vi "Device Sorter.vi"(0 "Mercury Ref":T3, 5 "Devices":string[](array[string]), 11 "error in":errorcluster, 12 "ISOBUS address":T2=-1) -> (1 "Temp Dev Settings Array":T6[](array[typedef]), 2 "Heater Device Settings Array":T15[](array[typedef]), 3 "Aux Device Settings Array":T17[](array[typedef]) {"Signals"."% Open" min=0.0 max=100.0 step=0.1 format="%.4f"; "Signals"."Position" max=20.0 step=1.0 format="%.4f"; "Speed" max=7 step=1; "Gear" max=7 step=1; "Temp V Err" min=0.0 max=20.0 step=0.1; "Temp Err" min=0.0 max=20.0 step=0.1; "Scaling Factor" min=0.0 max=99.0 step=0.1; "Min Flow" min=0.0 max=20.0 step=0.1}, 4 "Mercury Ref Out":T3, 6 "Device_ref_Array":T3[](array[typedef]), 8 "Ch_type_index":i32[](array[numeric]), 10 "Device_Present?":bool[](array[boolean]), 13 "Level Device Settings Array":T19[](array[typedef]), 14 "Pressure Device Settings Array":T27[](array[typedef]), 15 "error out":errorcluster)   [LabVIEW 2013]
uses:
  <instrlib>/Mercury iXX/Public/Controls/Mercury Reference.ctl
  <instrlib>/Mercury iXX/Public/Controls/Comms Transport Layer.ctl
  <instrlib>/Mercury iXX/Private/Controls/Query Dynamic Reference.ctl
  <instrlib>/Mercury iXX/Public/Libraries/Temperature/Controls/Temperature Device (Read).ctl
  <instrlib>/Mercury iXX/Public/Controls/Manufacturing Data.ctl
  <instrlib>/Mercury iXX/Public/Libraries/Temperature/Controls/Temperature Sensor Type.ctl
  <instrlib>/Mercury iXX/Public/Libraries/Temperature/Controls/Excitation Cluster.ctl
  <instrlib>/Mercury iXX/Public/Libraries/Temperature/Controls/Excitation Type.ctl
  <instrlib>/Mercury iXX/Public/Libraries/Temperature/Controls/Calibration Cluster.ctl
  <instrlib>/Mercury iXX/Public/Libraries/Temperature/Controls/Calibration Interpolation.ctl
  <instrlib>/Mercury iXX/Public/Libraries/Temperature/Controls/Loop Cluster.ctl
  <instrlib>/Mercury iXX/Public/Libraries/Temperature/Controls/Temperature Signals Cluster.ctl
  <instrlib>/Mercury iXX/Public/Libraries/Heater/Controls/Heater Device (Read).ctl
  <instrlib>/Mercury iXX/Public/Libraries/Heater/Controls/Heater Signals Cluster.ctl
  <instrlib>/Mercury iXX/Public/Libraries/Auxiliary/Controls/AUX Device (Read).ctl
  <instrlib>/Mercury iXX/Public/Libraries/Auxiliary/Controls/AUX Signals (Read).ctl
  <instrlib>/Mercury iXX/Public/Libraries/Level Meter/Controls/Level Meter (Read).ctl
  <instrlib>/Mercury iXX/Public/Libraries/Level Meter/Controls/Nitrogen Configuration.ctl
  <instrlib>/Mercury iXX/Public/Libraries/Level Meter/Controls/Frequency Configuration.ctl
  <instrlib>/Mercury iXX/Public/Libraries/Level Meter/Controls/Signals.ctl
  <instrlib>/Mercury iXX/Public/Libraries/Level Meter/Controls/Helium Configuration.ctl
  <instrlib>/Mercury iXX/Public/Libraries/Level Meter/Controls/Resistance Configuration.ctl
  <instrlib>/Mercury iXX/Public/Libraries/Level Meter/Controls/Pre-Pulse.ctl
  <instrlib>/Mercury iXX/Public/Libraries/Level Meter/Controls/Pulse.ctl
  <instrlib>/Mercury iXX/Public/Libraries/Pressure/Controls/Pressure Device (Read).ctl
  <instrlib>/Mercury iXX/Public/Libraries/Pressure/Controls/Pressure Sensor Type.ctl
  <instrlib>/Mercury iXX/Public/Libraries/Pressure/Controls/Calibration Cluster.ctl
  <instrlib>/Mercury iXX/Public/Libraries/Pressure/Controls/Calibration Interpolation.ctl
  <instrlib>/Mercury iXX/Public/Libraries/Pressure/Controls/Loop Cluster.ctl
  <instrlib>/Mercury iXX/Public/Libraries/Pressure/Controls/Pressure Signals Cluster.ctl
  <instrlib>/Mercury iXX/Public/Controls/ISOBus Address.ctl
  <instrlib>/Mercury iXX/Public/Libraries/Temperature/Open/Open Temperature Device.vi
  <instrlib>/Mercury iXX/Public/Libraries/Temperature/Configuration/Read/Temperature Device (Read).vi
  <instrlib>/Mercury iXX/Public/Libraries/Heater/Open/Open Heater Device.vi
  <instrlib>/Mercury iXX/Public/Libraries/Heater/Configuration/Read/Heater Device (Read).vi
  <instrlib>/Mercury iXX/Public/Libraries/Auxiliary/Open/Open Auxiliary Device.vi
  <instrlib>/Mercury iXX/Public/Libraries/Auxiliary/Configuration/Read/Aux Device (Read).vi
  <instrlib>/Mercury iXX/Public/Libraries/Level Meter/Open/Open Level Meter Device.vi
  <instrlib>/Mercury iXX/Public/Libraries/Level Meter/Configuration/Read/Level Meter Device (Read).vi
  <instrlib>/Mercury iXX/Public/Libraries/Pressure/Open/Open Pressure Device.vi
  <instrlib>/Mercury iXX/Public/Libraries/Pressure/Configuration/Read/Pressure Device (Read).vi
  <instrlib>/Mercury iXX/Mercury iXX.lvlib
  <instrlib>/Mercury iXX/Public/Libraries/Temperature.lvlib
  <instrlib>/Mercury iXX/Public/Libraries/Heater.lvlib
  <instrlib>/Mercury iXX/Public/Libraries/Auxiliary.lvlib
  <instrlib>/Mercury iXX/Public/Libraries/Level Meter.lvlib
  <instrlib>/Mercury iXX/Public/Libraries/Pressure.lvlib
panel:
  in  "Tab Control":T1(tab)
  in  "Pres Dev":T27
  in  "LVL Dev":T19
  in  "Aux Dev":T17 {"Signals"."% Open" min=0.0 max=100.0 step=0.1 format="%.4f"; "Signals"."Position" max=20.0 step=1.0 format="%.4f"; "Speed" max=7 step=1; "Gear" max=7 step=1; "Temp V Err" min=0.0 max=20.0 step=0.1; "Temp Err" min=0.0 max=20.0 step=0.1; "Scaling Factor" min=0.0 max=99.0 step=0.1; "Min Flow" min=0.0 max=20.0 step=0.1}
  in  "Htr Dev Det":T15
  in  "Device Det":T6
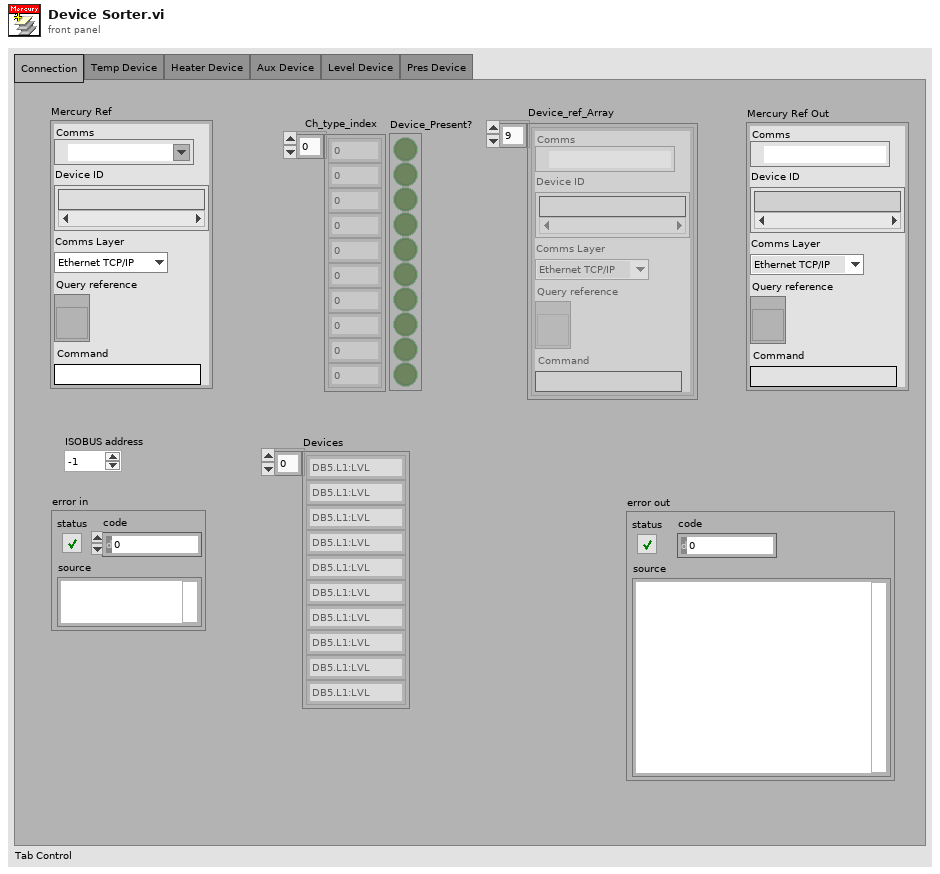
[diagram p1: front panel]
types:
  T1 = enum32{"Connection", "Temp Device", "Heater Device", "Aux Device", "Level Device", "Pres Device"}
  T2 = typedef "Mercury iXX.lvlib/ISOBus Address.ctl" = i32
  T3 = typedef "Mercury iXX.lvlib/Mercury Reference.ctl" = cluster{"Comms":refnum<visa-resource-name>, "Device ID":string[], "Comms Layer":T4, "Command":string, "Query reference":T5}
  T4 = typedef "Mercury iXX.lvlib/Comms Transport Layer.ctl" = enum16{"Ethernet TCP/IP", "USB", "ISOBus - RS-232", "GPIB"}
  T5 = typedef "Mercury iXX.lvlib/Query Dynamic Reference.ctl" = refnum<vi>
  T6 = typedef "Mercury iXX.lvlib/Temperature.lvlib/Temperature Device (Read).ctl" = cluster{"Manufacturing":T7, "Temperature Sensor Type":T8, "Excitation":T9, "Calibration":T11, "Control Loop":T13, "Temperature Signals":T14, "Nickname":string, "Status":string}
  T7 = typedef "Mercury iXX.lvlib/Manufacturing Data.ctl" = cluster{"Hardware Version":string, "Firmware Version":string, "Serial Number":string}
  T8 = typedef "Mercury iXX.lvlib/Temperature.lvlib/Temperature Sensor Type.ctl" = string
  T9 = typedef "Mercury iXX.lvlib/Temperature.lvlib/Excitation Cluster.ctl" = cluster{"Excitation Type":T10, "Magnitude":string}
  T10 = typedef "Mercury iXX.lvlib/Temperature.lvlib/Excitation Type.ctl" = string
  T11 = typedef "Mercury iXX.lvlib/Temperature.lvlib/Calibration Cluster.ctl" = cluster{"Filename":string, "Interpolation":T12, "Scaling Factor":string, "Offset Factor":string, "Hot Limit":string, "Cold Limit":string, "Last Calibration":string, "Reference":string}
  T12 = typedef "Mercury iXX.lvlib/Temperature.lvlib/Calibration Interpolation.ctl" = string
  T13 = typedef "Mercury iXX.lvlib/Temperature.lvlib/Loop Cluster.ctl" = cluster{"Heater":string, "Auxiliary":string, "Heater Auto":string, "Percentage Heat":string, "Temperature Set Point":string, "PID Auto (from file)":string, "P Value":string, "I Value":string, "D Value":string, "Auto PID Table Filename":string, "Flow Auto":string, "Target Heater Table":string, "Sweep mode":string, "Sweep Table Filename":string, "Percentage Flow":string}
  T14 = typedef "Mercury iXX.lvlib/Temperature.lvlib/Temperature Signals Cluster.ctl" = cluster{"Voltage":string, "Current":string, "Power":string, "Resistance":string, "Temperature":string, "Sensitivity":string, "Reference":string}
  T15 = typedef "Mercury iXX.lvlib/Heater.lvlib/Heater Device (Read).ctl" = cluster{"Manufacturing":T7, "Nickname":string, "Voltage Limit":string, "Nominal Resistance":string, "Maximum Power":string, "Heater Signals":T16, "Status":string}
  T16 = typedef "Mercury iXX.lvlib/Heater.lvlib/Heater Signals Cluster.ctl" = cluster{"Voltage":string, "Current":string, "Power":string}
  T17 = typedef "Mercury iXX.lvlib/Auxiliary.lvlib/AUX Device (Read).ctl" = cluster{"Manufacturing":T7, "Min Flow":dbl, "Scaling Factor":dbl, "Temp Err":dbl, "Temp V Err":dbl, "Gear":u32, "Speed":u32, "Signals":T18, "Nickname":string, "Status":string}
  T18 = typedef "Mercury iXX.lvlib/Auxiliary.lvlib/AUX Signals (Read).ctl" = cluster{"Position":dbl, "% Open":dbl, "I0":string, "I1":string, "I2":string, "I3":string, "O0":string, "O1":string, "O2":string, "O3":string}
  T19 = typedef "Mercury iXX.lvlib/Level Meter.lvlib/Level Meter (Read).ctl" = cluster{"Manufacturing":T7, "Nitrogen Configuration":T20, "Signals":T22, "Nickname":string, "Status":string, "Helium Configuration":T23}
  T20 = typedef "Mercury iXX.lvlib/Level Meter.lvlib/Nitrogen Configuration.ctl" = cluster{"Frequency Configuration":T21, "Pulse Period":dbl}
  T21 = typedef "Mercury iXX.lvlib/Level Meter.lvlib/Frequency Configuration.ctl" = cluster{"Freq 0%":dbl, "Freq 100%":dbl}
  T22 = typedef "Mercury iXX.lvlib/Level Meter.lvlib/Signals.ctl" = cluster{"Helium Signals":cluster{"Resistance":dbl, "Level":dbl}, "Nitrogen Signals":cluster{"Count":dbl, "Freq":dbl, "Level":dbl}}
  T23 = typedef "Mercury iXX.lvlib/Level Meter.lvlib/Helium Configuration.ctl" = cluster{"Resistance Configuration":T24, "Pre-Pulse":T25, "Pulse":T26}
  T24 = typedef "Mercury iXX.lvlib/Level Meter.lvlib/Resistance Configuration.ctl" = cluster{"Res 0%":dbl, "Res 100%":dbl}
  T25 = typedef "Mercury iXX.lvlib/Level Meter.lvlib/Pre-Pulse.ctl" = cluster{"Magnitude":dbl, "Duration":dbl}
  T26 = typedef "Mercury iXX.lvlib/Level Meter.lvlib/Pulse.ctl" = cluster{"Magnitude":dbl, "Duration":dbl, "Delay":dbl}
  T27 = typedef "Mercury iXX.lvlib/Pressure.lvlib/Pressure Device (Read).ctl" = cluster{"Manufacturing":T7, "Temperature Sensor Type":T28, "Calibration":T29, "Control Loop":T31, "Pressure Signals":T32, "Nickname":string, "Status":string}
  T28 = typedef "Mercury iXX.lvlib/Pressure.lvlib/Pressure Sensor Type.ctl" = string
  T29 = typedef "Mercury iXX.lvlib/Pressure.lvlib/Calibration Cluster.ctl" = cluster{"Filename":string, "Interpolation":T30, "Scaling Factor":string, "Offset Factor":string, "High Limit":string, "Low Limit":string, "Last Calibration":string}
  T30 = typedef "Mercury iXX.lvlib/Pressure.lvlib/Calibration Interpolation.ctl" = string
  T31 = typedef "Mercury iXX.lvlib/Pressure.lvlib/Loop Cluster.ctl" = cluster{"Heater":string, "Auxiliary":string, "Heater Auto":string, "Percentage Heat":string, "Pressure Set Point":string, "PID Auto (from file)":string, "P Value":string, "I Value":string, "D Value":string, "Auto PID Table Filename":string, "Flow Auto":string, "Target Heater Table":string, "Sweep mode":string, "Sweep Table Filename":string, "Percentage Flow":string}
  T32 = typedef "Mercury iXX.lvlib/Pressure.lvlib/Pressure Signals Cluster.ctl" = cluster{"Voltage":string, "Current":string, "Power":string, "Pressure":string}
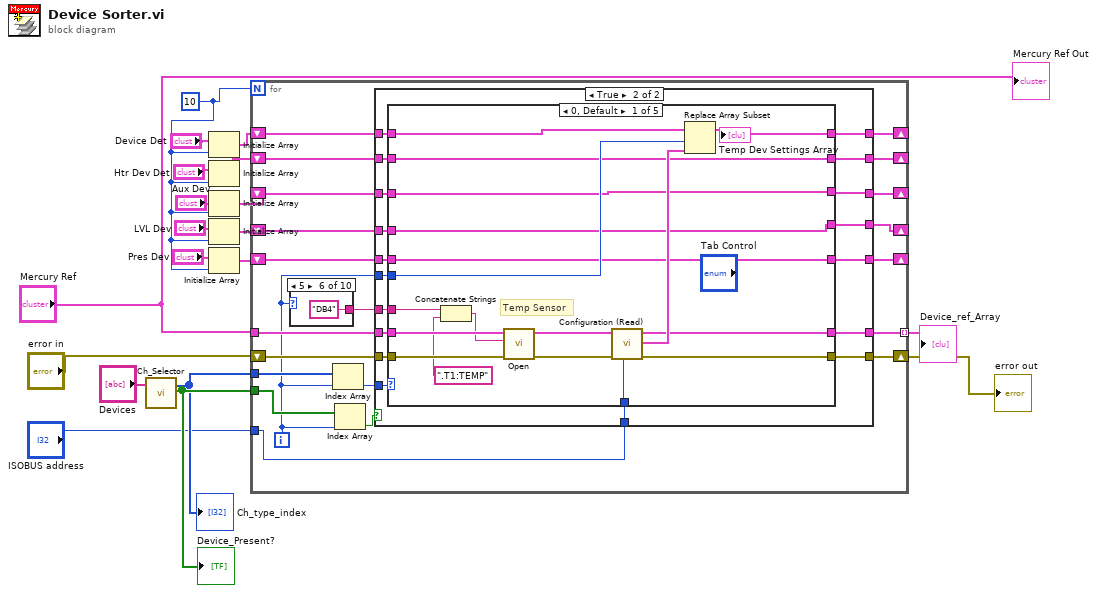
[diagram p0: block diagram]
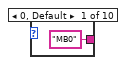
[diagram p2: hidden frame]
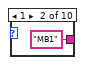
[diagram p3: hidden frame]
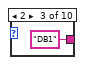
[diagram p4: hidden frame]
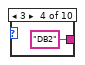
[diagram p5: hidden frame]
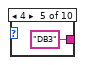
[diagram p6: hidden frame]
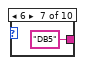
[diagram p7: hidden frame]
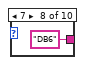
[diagram p8: hidden frame]
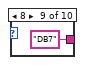
[diagram p9: hidden frame]
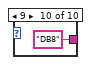
[diagram p10: hidden frame]
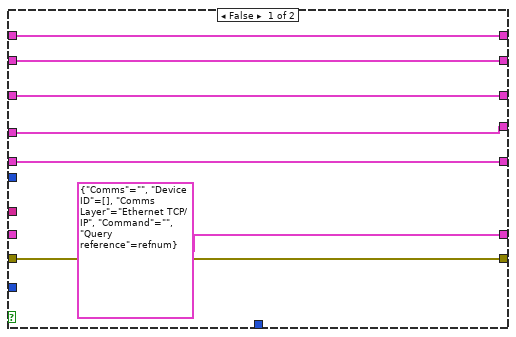
[diagram p11: hidden frame]
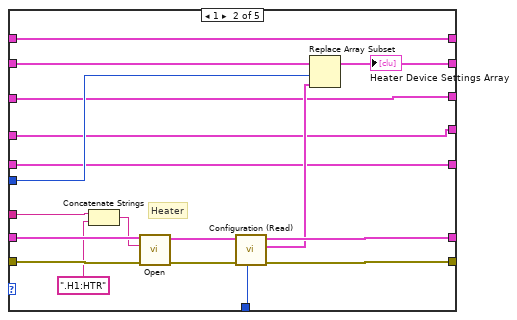
[diagram p12: hidden frame]
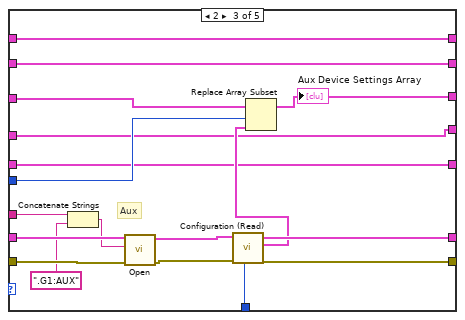
[diagram p13: hidden frame]
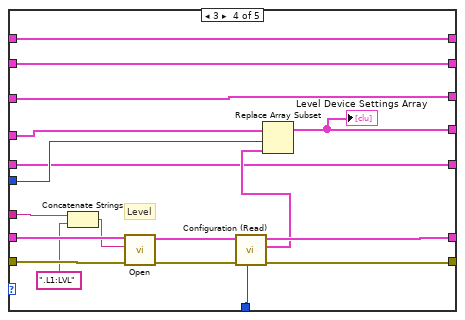
[diagram p14: hidden frame]
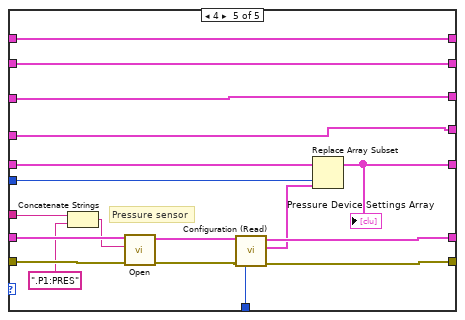
[diagram p15: hidden frame]
diagram:
  w9 = 10
  n1 = call <instrlib>:"Ch_Selector.vi"("Devices"="Devices") -> ("Ch_type_index"=w18:i32[], "Device_Present?"=w19:bool[])
  "Ch_type_index" <- w18
  "Device_Present?" <- w19
  n2 = Initialize Array("Device Det", w9) -> (w14:T6[])
  n3 = Initialize Array("Htr Dev Det", w9) -> (w12:T15[])
  n4 = Initialize Array("Aux Dev", w9) -> (w10:T17[])
  n5 = Initialize Array("LVL Dev", w9) -> (w7:T19[])
  n6 = Initialize Array("Pres Dev", w9) -> (w5:T27[])
  n7 = for {
    N: w9 -> [_]
    tunnel: "Mercury Ref" -> [w40]
    tunnel: [w39] -> w17 mode=indexing
    tunnel: w18 -> [w38]
    tunnel: w19 -> [w37]
    shift-right: [w32] -> w16
    shift-left: "error in" -> [w33]
    shift-right: [w30] -> _
    shift-left: w14 -> [w29]
    shift-right: [w28] -> _
    shift-left: w12 -> [w27]
    tunnel: "ISOBUS address" -> [w20]
    shift-right: [w26] -> _
    shift-left: w10 -> [w25]
    shift-right: [w23] -> _
    shift-left: w7 -> [w24]
    shift-right: [w22] -> _
    shift-left: w5 -> [w21]
    i -> [w31]
    n8 = case shown="5" w31 {
      tunnel: ["MB0" "MB1" "DB1" "DB2" "DB3" "DB4" "DB5" "DB6" "DB7" "DB8"] -> w34
      frame 0, Default {
      }
      frame 1 {
      }
      frame 2 {
      }
      frame 3 {
      }
      frame 4 {
      }
      frame 5 {
      }
      frame 6 {
      }
      frame 7 {
      }
      frame 8 {
      }
      frame 9 {
      }
    }
    n9 = Index Array(array=w38, index=w31) -> (element=w35:i32)
    n10 = Index Array(array=w37, index=w31) -> (element=w36:bool)
    n11 = case shown="True" w36 {
      tunnel: w40 -> [_ w75]
      tunnel: w33 -> [w56 w74]
      tunnel: [T3 {"Comms"="", "Device ID"=[], "Comms Layer"=enum."Ethernet TCP/IP", "Command"="", "Query reference"=refnum} ("Mercury Reference Out") w73] -> w39
      tunnel: [w56 w72] -> w32
      tunnel: w35 -> [_ w71]
      tunnel: w34 -> [_ w70]
      tunnel: w31 -> [_ w69]
      tunnel: [w55 w67] -> w30
      tunnel: w29 -> [w55 w68]
      tunnel: [w54 w66] -> w28
      tunnel: w27 -> [w54 w65]
      tunnel: w20 -> [_ w64]
      tunnel: [w53 w63] -> w26
      tunnel: w25 -> [w53 w62]
      tunnel: w24 -> [w52 w61]
      tunnel: [w52 w60] -> w23
      tunnel: [w51 w59] -> w22
      tunnel: w21 -> [w51 w58]
      frame False {
      }
      frame True {
        n12 = case shown="0, Default" w71 {
          tunnel: w74 -> [w93 w111 w129 w147 w165]
          tunnel: w75 -> [w92 w110 w128 w146 w164]
          tunnel: [w83 w104 w120 w138 w156] -> w73
          tunnel: [w82 w103 w119 w137 w155] -> w72
          tunnel: w70 -> [w91 w107 w125 w143 w161]
          tunnel: w69 -> [w86 w102 w117 w132 w150]
          tunnel: [w81 w100 w124 w142 w160] -> w67
          tunnel: w68 -> [w84 w100 w124 w142 w160]
          tunnel: [w80 w98 w123 w141 w159] -> w66
          tunnel: w65 -> [w80 w99 w123 w141 w159]
          tunnel: w64 -> [w79 w97 w118 w136 w154]
          tunnel: [w78 w96 w115 w135 w153] -> w63
          tunnel: w62 -> [w78 w96 w114 w135 w153]
          tunnel: w61 -> [w77 w95 w113 w133 w152]
          tunnel: [w77 w95 w113 w131 w152] -> w60
          tunnel: [w76 w94 w112 w130 w148] -> w59
          tunnel: w58 -> [w76 w94 w112 w130 w149]
          frame 0, Default {
            # "Temp Sensor"
            n13 = Concatenate Strings(w91, ".T1:TEMP" ("Device Identifier")) -> (w89:string)
            n14 = call-poly <instrlib>:"Open.vi"("error in (no error)"=w93, "Device Identifier"=w89, "Mercury Reference In"=w92) -> ("error out"=w88:errorcluster, "Mercury Reference Out"=w87:T3)  [unwired: 1 in, 6 out]
            n15 = call-poly <instrlib>:"Configuration (Read).vi"("ISOBUS address"=w79, "error in"=w88, "Mercury Reference In"=w87) -> ("error out"=w82:errorcluster, "Device Details"=w85:T6, "Mercury Reference Out"=w83:T3)  [unwired: 6 out]
            n16 = Replace Array Subset(array=w84, new element=w85, index=w86) -> (w81:T6[])
            "Temp Dev Settings Array" <- w81
          }
          frame 1 {
            # "Heater"
            n17 = Concatenate Strings(w107, ".H1:HTR" ("Device Identifier")) -> (w108:string)
            n18 = call-poly <instrlib>:"Open.vi"("error in (no error)"=w111, "Device Identifier"=w108, "Mercury Reference In"=w110) -> ("error out"=w106:errorcluster, "Mercury Reference Out"=w105:T3)  [unwired: 7 in]
            n19 = call-poly <instrlib>:"Configuration (Read).vi"("ISOBUS address"=w97, "error in"=w106, "Mercury Reference In"=w105) -> ("error out"=w103:errorcluster, "Device Details"=w101:T15, "Mercury Reference Out"=w104:T3)  [unwired: 6 out]
            n20 = Replace Array Subset(array=w99, new element=w101, index=w102) -> (w98:T15[])
            "Heater Device Settings Array" <- w98
          }
          frame 2 {
            # "Aux"
            n21 = Concatenate Strings(w125, ".G1:AUX" ("Device Identifier")) -> (w126:string)
            n22 = call-poly <instrlib>:"Open.vi"("error in (no error)"=w129, "Device Identifier"=w126, "Mercury Reference In"=w128) -> ("error out"=w121:errorcluster, "Mercury Reference Out"=w122:T3)  [unwired: 7 out]
            n23 = call-poly <instrlib>:"Configuration (Read).vi"("ISOBUS address"=w118, "error in"=w121, "Mercury Reference In"=w122) -> ("error out"=w119:errorcluster, "Auxiliary Device Details"=w116:T17, "Mercury Reference Out"=w120:T3)  [unwired: 5 in, 1 out]
            n24 = Replace Array Subset(array=w114, new element=w116, index=w117) -> (w115:T17[])
            "Aux Device Settings Array" <- w115
          }
          frame 3 {
            # "Level"
            n25 = Concatenate Strings(w143, ".L1:LVL" ("Device Identifier")) -> (w144:string)
            n26 = call-poly <instrlib>:"Open.vi"("error in (no error)"=w147, "Device Identifier"=w144, "Mercury Reference In"=w146) -> ("error out"=w139:errorcluster, "Mercury Reference Out"=w140:T3)  [unwired: 7 out]
            n27 = call-poly <instrlib>:"Configuration (Read).vi"("ISOBUS address"=w136, "error in"=w139, "Mercury Reference In"=w140) -> ("error out"=w137:errorcluster, "LVL Device Settings"=w134:T19, "Mercury Reference Out"=w138:T3)  [unwired: 5 in, 1 out]
            n28 = Replace Array Subset(array=w133, new element=w134, index=w132) -> (w131:T19[])
            "Level Device Settings Array" <- w131
          }
          frame 4 {
            # "Pressure sensor"
            n29 = Concatenate Strings(w161, ".P1:PRES" ("Device Identifier")) -> (w162:string)
            n30 = call-poly <instrlib>:"Open.vi"("error in (no error)"=w165, "Device Identifier"=w162, "Mercury Reference In"=w164) -> ("error out"=w157:errorcluster, "Mercury Reference Out"=w158:T3)  [unwired: 7 out]
            n31 = call-poly <instrlib>:"Configuration (Read).vi"("ISOBUS address"=w154, "error in"=w157, "Mercury Reference In"=w158) -> ("error out"=w155:errorcluster, "Device Details"=w151:T27, "Mercury Reference Out"=w156:T3)  [unwired: 5 in, 1 out]
            n32 = Replace Array Subset(array=w149, new element=w151, index=w150) -> (w148:T27[])
            "Pressure Device Settings Array" <- w148
          }
        }
      }
    }
  }
  "Device_ref_Array" <- w17
  "error out" <- w16
  "Mercury Ref Out" <- "Mercury Ref"
